vi "ECC_v3.vi"() -> ()   [LabVIEW 2019]
uses:
  state_machine.ctl
  <vilib>/DAQmx/write.llb/DAQmx Write (Analog Wfm 1Chan NSamp).vi
  <vilib>/DAQmx/create/channels.llb/DAQmx Create Channel (AO-Voltage-Basic).vi
  <vilib>/DAQmx/configure/timing.llb/DAQmx Timing (Use Waveform).vi
  <vilib>/DAQmx/miscellaneous.llb/DAQmx Fill In Error Info.vi
panel:
  in  "Use_DAC":bool
  out "AMP_status":bool
  in  "APS/APM":bool=TRUE
  in  "AMP address":tag="Dev1/port0/line0"
  in  "R&S/5181":bool=TRUE
  out "Pause, s":i32
  out "APS_off_status":bool=TRUE
  out "R&S_off_status":bool=TRUE
  out "Countdown":u32
  in  "Rep_delay":u32
  in  "Finite/Continuous":bool
  in  "ResumeSweep":bool
  in  "PauseSweep":bool
  in  "RF_off_rep":bool=TRUE
  in  "RF_off_set":bool
  in  "RF_off_cycle":bool
  in  "APS_off_rep":bool=TRUE
  in  "APS_off_set":bool
  in  "APS_off_cycle":bool
  in  "AbortSweep":bool
  in  "Check APS":bool
  in  "ON/OFF_APS":bool
  in  "Check R&S":bool
  in  "ON/OFF_RF":bool
  in  "Use_APS":bool
  out "DAC_status":bool
  out "RF_status":bool
  out "i_Current_repetition":i32
  out "N_Cycles_Created":i32
  out "i_Current_cycle":i32
  in  "M_repetitions":i32 min=0
  in  "Set_of_Cycles":T1(array[cluster])=[{"On/Off"=TRUE, "f0, MHz"=32.5, "fm, kHz"=1000, "A, mV"=20, "Waveform"=enum."triangle", "N_steps"=500, "T_sweep, s"=10.0, "N_sweeps"=5, "End_Wait, s"=0}, {"On/Off"=TRUE, "f0, MHz"=62.7, "fm, kHz"=400, "A, mV"=10, "Waveform"=enum."triangle", "N_steps"=500, "T_sweep, s"=10.0, "N_sweeps"=5, "End_Wait, s"=0}] {"End_Wait, s" step=1; "N_sweeps" min=0 step=1; "T_sweep, s" min=0.0 step=0.001 format="%#_6f"; "N_steps" min=0 step=1; "fm, kHz" step=1; "f0, MHz" min=0.0 step=0.001 format="%#_6f"}
  out "APS_status":bool
  in  "APS address":refnum<visa-resource-name>="COM3"
  in  "Init Devices":bool
  in  "Do Sweep":bool
  in  "Exit":bool
  in  "DAC channel":tag="Dev1/ao0"
  in  "RF address":string(combo)="19"
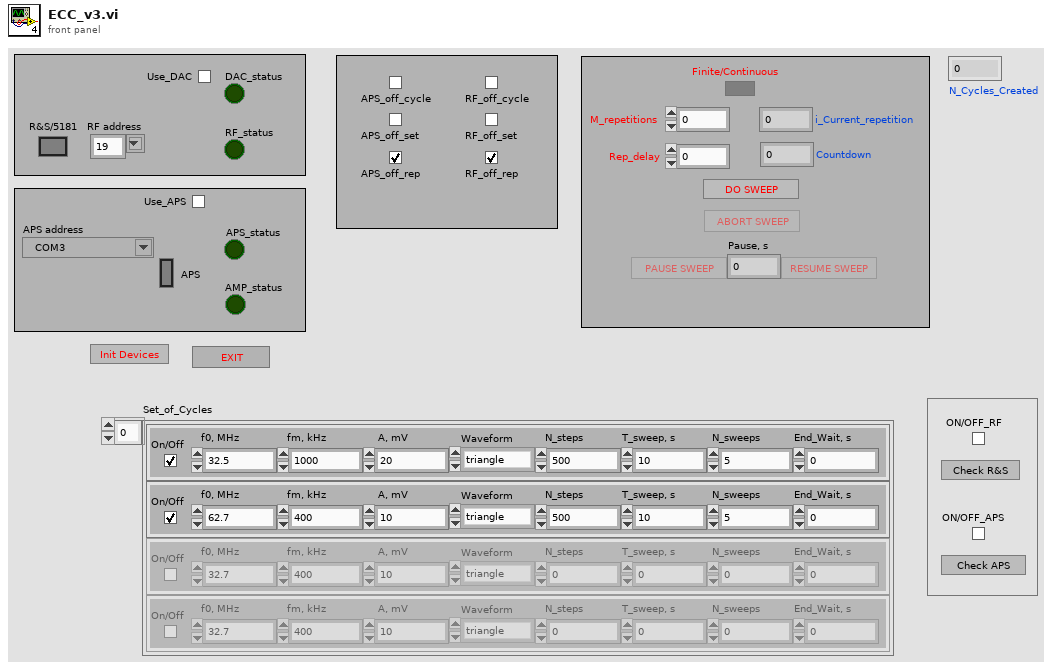
[diagram p1: front panel]
types:
  T1 = cluster{"On/Off":bool, "f0, MHz":dbl, "fm, kHz":i32, "A, mV":i32, "Waveform":enum16{"triangle", "saw_direct", "saw_invert", "sine"}, "N_steps":i32, "T_sweep, s":dbl, "N_sweeps":i32, "End_Wait, s":u32}[]
  T2 = typedef "state_machine.ctl" = enum16{"idle", "init_daq", "init_rf", "init_ps", "cycle_start", "get_wf", "rf_on", "rf_off", "rf_set", "ps_on", "ps_off", "daq_start", "daq_stop", "daq_wait", "daq_dt", "daq_v", "delay", "cycle_reset", "exit", "repetition_reset"}
  T3 = enum8{"Enabled", "Disabled", "Disabled and Grayed Out"}
  T4 = cluster{"On/Off":bool, "f0, MHz":dbl, "fm, kHz":i32, "A, mV":i32, "Waveform":enum16{"triangle", "saw_direct", "saw_invert", "sine"}, "N_steps":i32, "T_sweep, s":dbl, "N_sweeps":i32, "End_Wait, s":u32}
  T5 = enum16{"triangle", "saw_direct", "saw_invert", "sine"}
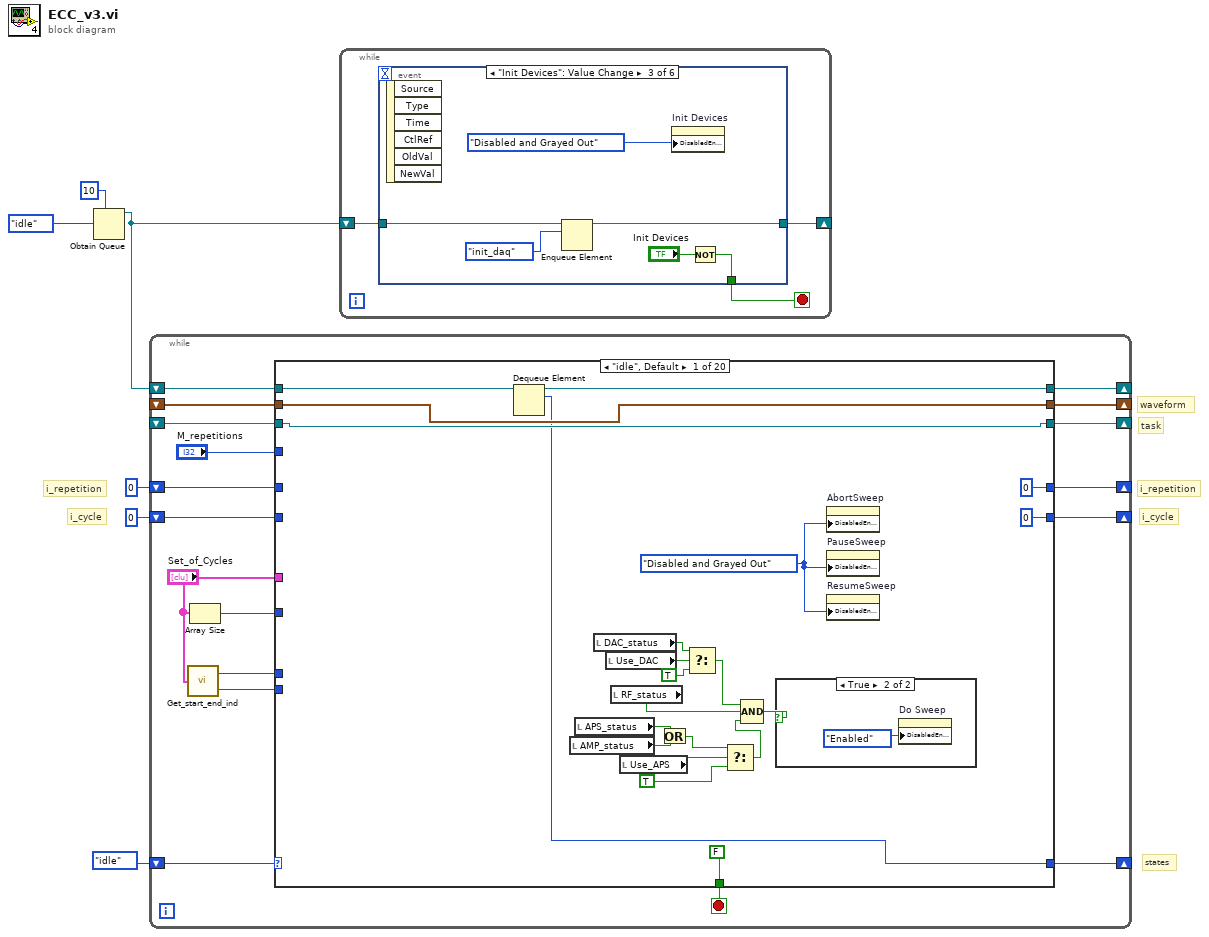
[diagram p0: block diagram]
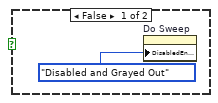
[diagram p2: hidden frame]
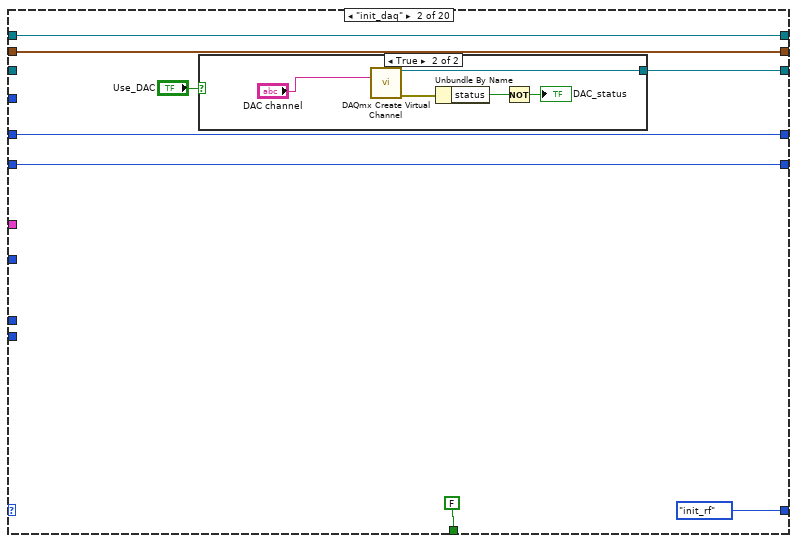
[diagram p3: hidden frame]
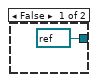
[diagram p4: hidden frame]
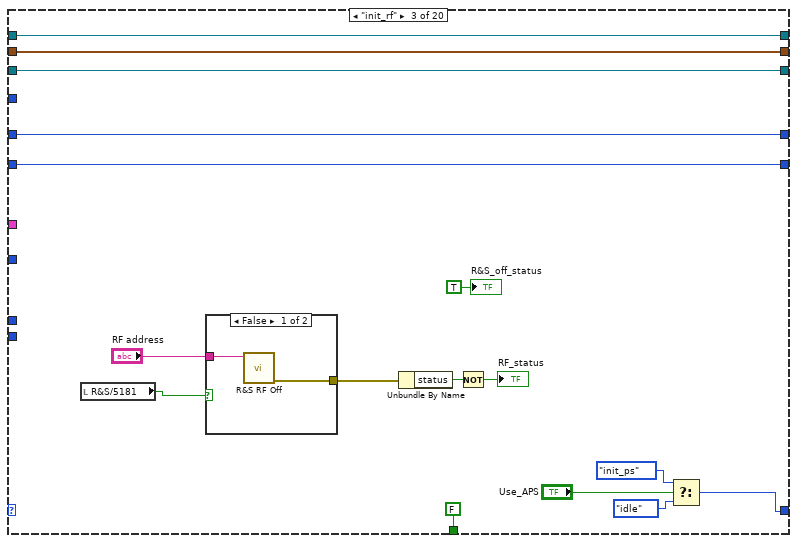
[diagram p5: hidden frame]
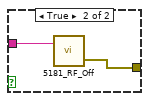
[diagram p6: hidden frame]
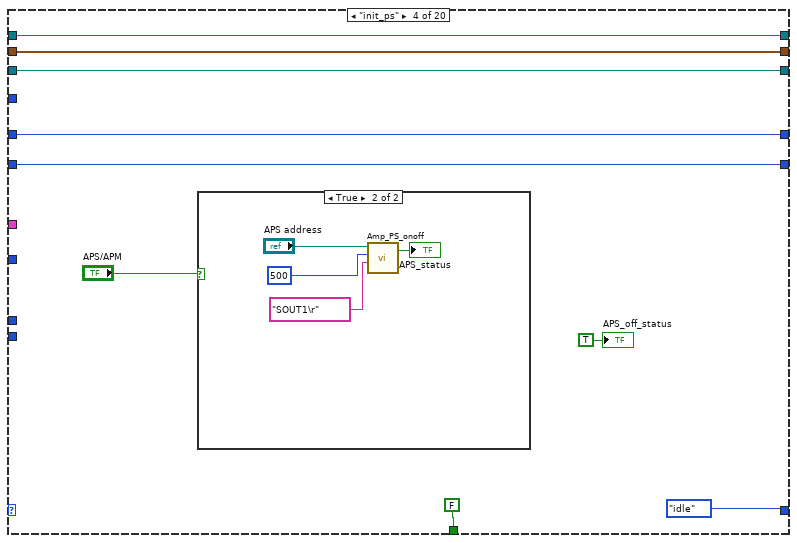
[diagram p7: hidden frame]
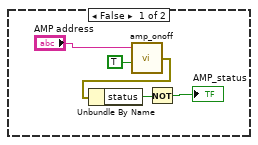
[diagram p8: hidden frame]
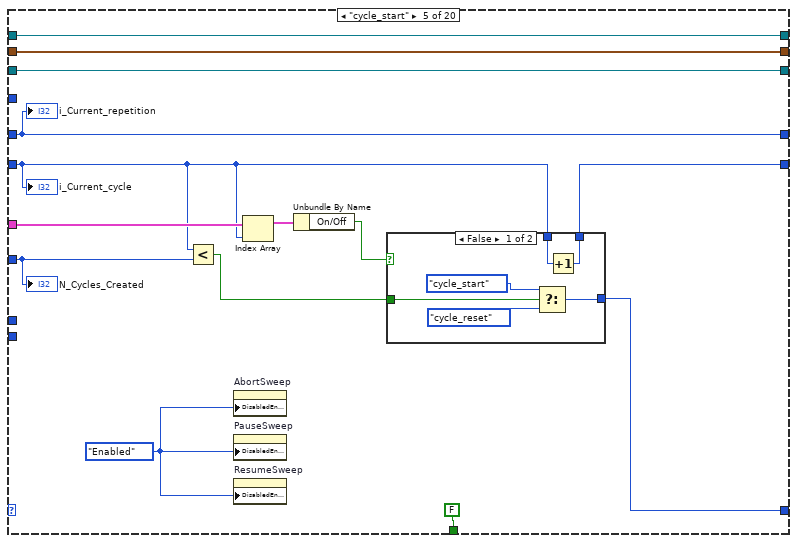
[diagram p9: hidden frame]
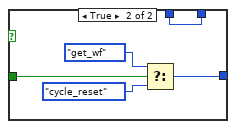
[diagram p10: hidden frame]
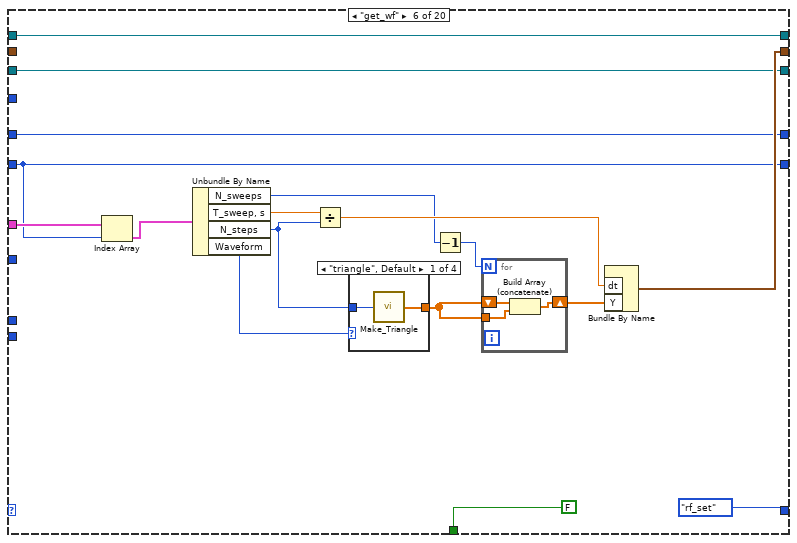
[diagram p11: hidden frame]
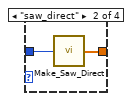
[diagram p12: hidden frame]
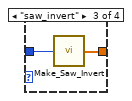
[diagram p13: hidden frame]
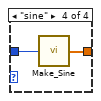
[diagram p14: hidden frame]
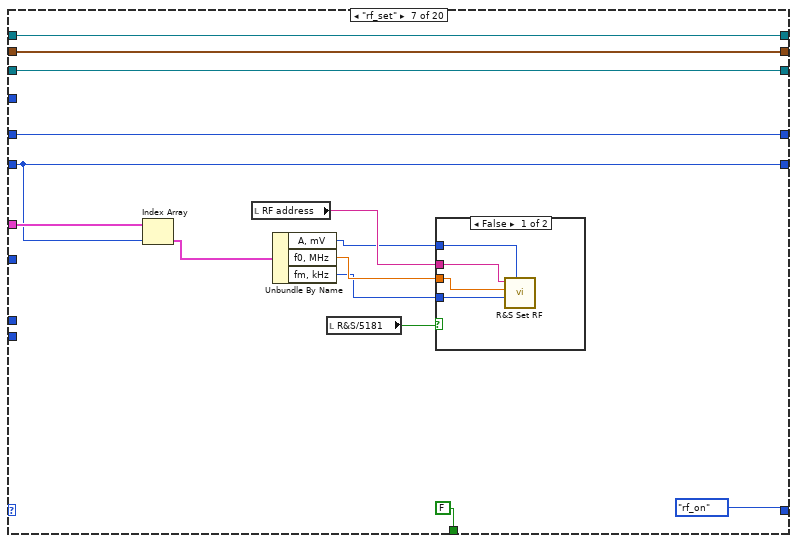
[diagram p15: hidden frame]
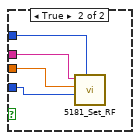
[diagram p16: hidden frame]
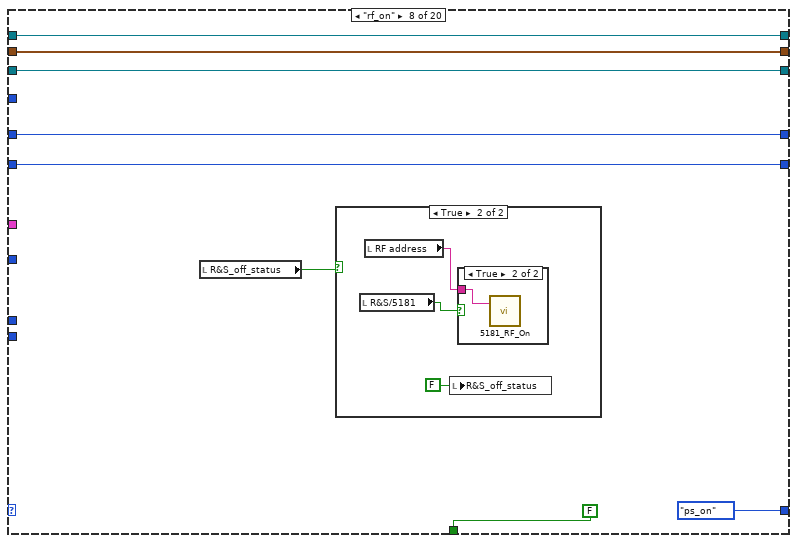
[diagram p17: hidden frame]
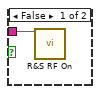
[diagram p19: hidden frame]
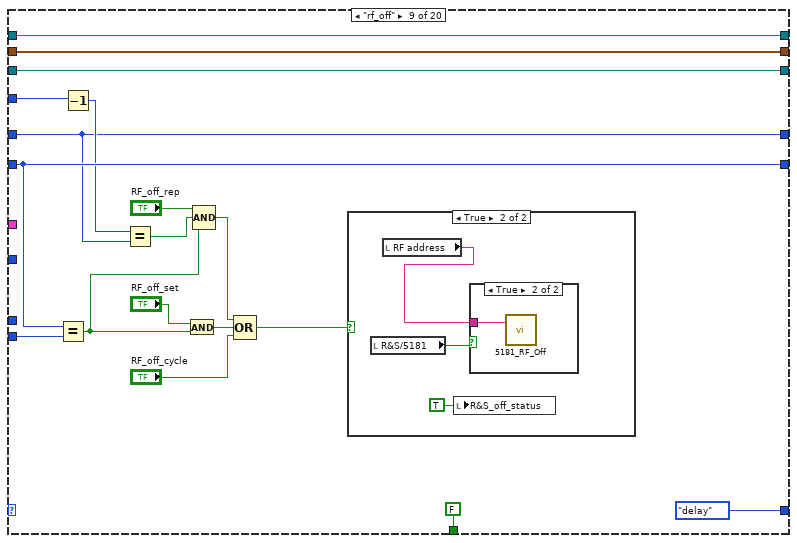
[diagram p20: hidden frame]
diagram:
  # "i_repetition"
  # "i_cycle"
  # "i_repetition"
  # "i_cycle"
  # "states"
  # "waveform"
  # "task"
  n1 = Obtain Queue(max queue size (-1, unlimited)=10, element data type=state_machine."idle") -> (queue out=w4:refnum<queue>)  [unwired: 3 in, 2 out]
  n2 = while {
    shift-right: [w19] -> _
    shift-left: state_machine."idle" -> [w24]
    shift-right: [w23] -> _
    shift-left: _ -> [w21]
    shift-right: [w22] -> _
    shift-left: _ -> [w20]
    shift-right: [w17] -> _
    shift-left: w4 -> [w18]
    shift-right: [w15] -> _
    shift-left: 0 -> [w14]
    shift-right: [w13] -> _
    shift-left: 0 -> [w12]
    stop <- w16 stop-if-true
    n3 = call "Get_start_end_ind.vi"("Set_of_Cycles"="Set_of_Cycles") -> ("start_ind"=w9:i32, "end_ind"=w8:i32)
    n4 = Array Size(array="Set_of_Cycles") -> (size(s)=w11:i32)
    n5 = case shown="\"idle\", Default" w24 {
      selector: w24 -> [_ _ _ _ _ _ _ _ _ _ _ _ _ _ _ _ _ _ w404 _]
      tunnel: [w45 w55 w77 w90 w103 w134 w163 w180 w203 w222 w243 w271 w283 w295 w307 w320 w336 w354 w401 w412] -> w23
      tunnel: "Set_of_Cycles" -> [_ _ _ _ w113 w141 w165 _ _ _ _ _ _ _ _ _ w333 _ _ _]
      tunnel: [w44 w54 w76 w89 w104 w135 w162 w181 w204 w221 w242 w270 w282 w294 w306 w321 w337 w353 w400 w413] -> w22
      tunnel: w21 -> [w45 _ w77 w90 w103 w134 w163 w180 w203 w222 w243 w272 w284 w296 w308 w322 w336 w354 w401 w412]
      tunnel: w20 -> [w44 w54 w76 w89 w104 _ w162 w181 w204 w221 w242 w270 w282 w294 w306 w321 w337 w353 w400 w413]
      tunnel: [w41 state_machine."init_rf" w67 state_machine."idle" w109 state_machine."rf_set" state_machine."rf_on" state_machine."ps_on" state_machine."delay" state_machine."daq_dt" state_machine."rf_off" state_machine."daq_wait" state_machine."ps_off" state_machine."daq_stop" state_machine."daq_v" state_machine."daq_start" state_machine."cycle_start" w352 w404 w408] -> w19
      tunnel: w18 -> [w43 w51 w74 w86 w102 w132 w160 w182 w205 w218 w239 w267 w279 w291 w303 w317 w338 w355 w403 w415]
      tunnel: [w42 w51 w74 w86 w102 w132 w160 w182 w205 w218 w239 w267 w279 w291 w303 w317 w338 w355 w403 w415] -> w17
      tunnel: [FALSE FALSE FALSE FALSE FALSE FALSE FALSE FALSE FALSE FALSE FALSE FALSE FALSE FALSE FALSE FALSE FALSE FALSE TRUE FALSE] -> w16
      tunnel: w11 -> [_ _ _ _ w105 _ _ _ _ _ _ _ _ _ _ _ _ _ _ _]
      tunnel: [0 w50 w73 w85 w108 w125 w158 w176 w199 w216 w237 w266 w278 w290 w302 w316 w328 0 w399 w414] -> w15
      tunnel: w14 -> [_ w50 w73 w85 w106 w125 w158 w176 w199 w216 w237 w266 w278 w290 w302 w316 w327 _ w399 w414]
      tunnel: [0 w49 w72 w84 w101 w127 w159 w179 w191 w217 w233 w265 w277 w289 w301 w315 w335 w349 w398 0] -> w13
      tunnel: w12 -> [_ w49 w72 w84 w101 w127 w159 w179 w191 w217 w233 w265 w277 w289 w301 w315 w335 w350 w398 _]
      tunnel: "M_repetitions" -> [_ _ _ _ _ _ _ _ w196 _ w235 _ _ _ _ _ _ w357 _ _]
      tunnel: w9 -> [_ _ _ _ _ _ _ _ _ _ _ _ _ _ _ _ _ _ _ _]
      tunnel: w8 -> [_ _ _ _ _ _ _ _ w200 _ w238 _ _ _ _ _ _ _ _ _]
      frame "idle", Default {
        w32 = T3."Disabled and Grayed Out" ("Disabled")
        n6 = Dequeue Element(queue=w43) -> (queue out=w42:refnum<queue>, element=w41:T2)  [unwired: 2 in, 2 out]
        n7 = local read "AMP_status"() -> (w30:bool)
        n8 = local read "APS_status"() -> (w31:bool)
        n9 = local read "DAC_status"() -> (w27:bool)
        n10 = local read "Use_DAC"() -> (w25:bool)
        n11 = local read "RF_status"() -> (w37:bool)
        n12 = local read "Use_APS"() -> (w36:bool)
        n13 = Or(x=w31, y=w30) -> (x .or. y?=w29:bool)
        n14 = Select(t=w27, s=w25, f=TRUE) -> (s? t:f=w28:bool)
        n15 = Select(t=w29, s=w36, f=TRUE) -> (s? t:f=w34:bool)
        n16 = Compound Arithmetic op=AND(w28, w37, w34) -> (w33:bool)
        n17 = case shown="True" w33 {
          frame False {
            n18 = property on="Do Sweep" class="Bool"("DisabledEnum"=T3."Disabled and Grayed Out" ("Disabled")) -> ()  [unwired: 2 in, 2 out]
          }
          frame True {
            n19 = property on="Do Sweep" class="Bool"("DisabledEnum"=T3."Enabled" ("Disabled")) -> ()  [unwired: 2 in, 2 out]
          }
        }
        n20 = property on="AbortSweep" class="Bool"("DisabledEnum"=w32) -> ()  [unwired: 2 in, 2 out]
        n21 = property on="PauseSweep" class="Bool"("DisabledEnum"=w32) -> ()  [unwired: 2 in, 2 out]
        n22 = property on="ResumeSweep" class="Bool"("DisabledEnum"=w32) -> ()  [unwired: 2 in, 2 out]
      }
      frame "init_daq" {
        n23 = case shown="True" "Use_DAC" {
          tunnel: [refnum<k21> refnum ("task out") w60] -> w55
          frame False {
          }
          frame True {
            n24 = call-poly <vilib>:"DAQmx Create Virtual Channel.vi"("physical channels"="DAC channel") -> ("task out"=w60:refnum<k21>, "error out"=w59:errorcluster)  [unwired: 13 in]
            n25 = Unbundle By Name(w59) -> ("status"=w58:bool)
            n26 = Not(x=w58) -> (.not. x?=→"DAC_status":bool)
          }
        }
      }
      frame "init_rf" {
        n27 = local read "R&S/5181"() -> (w62:bool)
        n28 = case shown="False" w62 {
          tunnel: "RF address" -> [w79 w81]
          tunnel: [w78 w80] -> w63
          frame False {
            n29 = call "R&S RF Off.vi"("address"=w79) -> ("error out"=w78:errorcluster)  [unwired: 5 in, 1 out]
          }
          frame True {
            n30 = call "5181_RF_Off.vi"("address"=w81) -> ("error out"=w80:errorcluster)  [unwired: 1 in, 1 out]
          }
        }
        n31 = Unbundle By Name(w63) -> ("status"=w70:bool)
        n32 = Not(x=w70) -> (.not. x?=→"RF_status":bool)
        n33 = Select(t=state_machine."init_ps", s="Use_APS", f=state_machine."idle") -> (s? t:f=w67:T2)
        "R&S_off_status" <- TRUE ("R&S_off_status")
      }
      frame "init_ps" {
        n34 = case shown="True" "APS/APM" {
          frame False {
            n35 = call "amp_onoff.vi"("amp_onoff"=TRUE, "AMP address"="AMP address") -> ("error out"=w93:errorcluster)  [unwired: 1 in]
            n36 = Unbundle By Name(w93) -> ("status"=w94:bool)
            n37 = Not(x=w94) -> (.not. x?=→"AMP_status":bool)
          }
          frame True {
            n38 = call "Amp_PS_onoff.vi"("On/Off Control"="SOUT1\r", "delay before read (ms)"=u32 500, "Amp PS address"="APS address") -> ("status"=→"APS_status":bool)  [unwired: 1 in, 1 out]
          }
        }
        "APS_off_status" <- TRUE ("APS_off_status")
      }
      frame "cycle_start" {
        w100 = T3."Enabled" ("Disabled")
        n39 = Less?(x=w106, y=w105) -> (x < y?=w110:bool)
        n40 = property on="AbortSweep" class="Bool"("DisabledEnum"=w100) -> ()  [unwired: 2 in, 2 out]
        n41 = property on="PauseSweep" class="Bool"("DisabledEnum"=w100) -> ()  [unwired: 2 in, 2 out]
        n42 = property on="ResumeSweep" class="Bool"("DisabledEnum"=w100) -> ()  [unwired: 2 in, 2 out]
        n43 = Index Array(array=w113, index=w106) -> (element=w112:T4)
        n44 = Unbundle By Name(w112) -> ("On/Off"=w111:bool)
        n45 = case shown="False" w111 {
          tunnel: w110 -> [w117 w123]
          tunnel: [w114 w122] -> w109
          tunnel: w106 -> [w119 w120]
          tunnel: [w118 w120] -> w108
          frame False {
            n46 = Select(t=state_machine."cycle_start", s=w117, f=state_machine."cycle_reset") -> (s? t:f=w114:T2)
            n47 = Increment(x=w119) -> (x+1=w118:i32)
          }
          frame True {
            n48 = Select(t=state_machine."get_wf", s=w123, f=state_machine."cycle_reset") -> (s? t:f=w122:T2)
          }
        }
        "N_Cycles_Created" <- w105
        "i_Current_cycle" <- w106
        "i_Current_repetition" <- w101
      }
      frame "get_wf" {
        n49 = Index Array(array=w141, index=w125) -> (element=w140:T4)
        n50 = Unbundle By Name(w140) -> ("N_sweeps"=w131:i32, "T_sweep, s"=w129:dbl, "N_steps"=w128:i32, "Waveform"=w130:T5)
        n51 = Divide(x=w129, y=w128) -> (x/y=w137:dbl)
        n52 = case shown="\"triangle\", Default" w130 {
          tunnel: w128 -> [w146 w148 w150 w152]
          tunnel: [w145 w147 w149 w151] -> w138
          frame "triangle", Default {
            n53 = call "Make_Triangle.vi"("N_steps_1"=w146) -> ("TriangleWaveform"=w145:dbl[])
          }
          frame "saw_direct" {
            n54 = call "Make_Saw_Direct.vi"("N_steps_1"=w148) -> ("SawDirectWaveform"=w147:dbl[])
          }
          frame "saw_invert" {
            n55 = call "Make_Saw_Invert.vi"("N_steps_1"=w150) -> ("SawInvertWaveform"=w149:dbl[])
          }
          frame "sine" {
            n56 = call "Make_Sine.vi"("N_steps_1"=w152) -> ("SineWaveform"=w151:dbl[])
          }
        }
        n57 = Decrement(x=w131) -> (x-1=w136:i32)
        n58 = for {
          N: w136 -> [_]
          shift-right: [w142] -> w139
          shift-left: w138 -> [w144]
          tunnel: w138 -> [w143]
          n59 = Build Array (concatenate)(w144, w143) -> (w142:dbl[])
        }
        n60 = Bundle By Name("dt"=w137, "Y"=w139) -> (w135:waveform(dbl))  [unwired: 1 in]
      }
      frame "rf_set" {
        n61 = Index Array(array=w165, index=w158) -> (element=w164:T4)
        n62 = local read "RF address"() -> (w166:string)
        n63 = Unbundle By Name(w164) -> ("A, mV"=w157:i32, "f0, MHz"=w156:dbl, "fm, kHz"=w155:i32)
        n64 = local read "R&S/5181"() -> (w153:bool)
        n65 = case shown="False" w153 {
          tunnel: w166 -> [w170 w174]
          tunnel: w157 -> [w169 w173]
          tunnel: w156 -> [w168 w172]
          tunnel: w155 -> [w167 w171]
          frame False {
            n66 = call "R&S Set RF.vi"("amplitude (mV)"=w169, "modulation (kHz)"=w167, "center frequency (MHz)"=w168, "address"=w170) -> ()  [unwired: 3 in, 2 out]
          }
          frame True {
            n67 = call "5181_Set_RF.vi"("address"=w174, "center frequency (MHz)"=w172, "modulation (kHz)"=w171, "amplitude (mV)"=w173) -> ()  [unwired: 1 in, 2 out]
          }
        }
      }
      frame "rf_on" {
        n68 = local read "R&S_off_status"() -> (w175:bool)
        n69 = case shown="True" w175 {
          frame False {
          }
          frame True {
            n70 = local read "R&S/5181"() -> (w183:bool)
            n71 = local read "RF address"() -> (w185:string)
            n72 = local write "R&S_off_status"(FALSE ("R&S_off_status")) -> ()
            n73 = case shown="True" w183 {
              tunnel: w185 -> [w186 w187]
              frame False {
                n74 = call "R&S RF On.vi"("address"=w186) -> ()  [unwired: 5 in, 2 out]
              }
              frame True {
                n75 = call "5181_RF_On.vi"("address"=w187) -> ()  [unwired: 1 in, 2 out]
              }
            }
          }
        }
      }
      frame "rf_off" {
        n76 = Equal?(x=w199, y=w200) -> (x = y?=w188:bool)
        n77 = Decrement(x=w196) -> (x-1=w192:i32)
        n78 = Equal?(x=w192, y=w191) -> (x = y?=w189:bool)
        n79 = And(x="RF_off_set", y=w188) -> (x .and. y?=w195:bool)
        n80 = Compound Arithmetic op=AND("RF_off_rep", w189, w188) -> (w193:bool)
        n81 = Compound Arithmetic op=OR(w193, w195, "RF_off_cycle") -> (w197:bool)
        n82 = case shown="True" w197 {
          frame False {
          }
          frame True {
            n83 = local read "R&S/5181"() -> (w206:bool)
            n84 = local read "RF address"() -> (w208:string)
            n85 = local write "R&S_off_status"(TRUE ("R&S_off_status")) -> ()
            n86 = case shown="True" w206 {
              tunnel: w208 -> [w209 w210]
              frame False {
                n87 = call "R&S RF Off.vi"("address"=w209) -> ()  [unwired: 5 in, 2 out]
              }
              frame True {
                n88 = call "5181_RF_Off.vi"("address"=w210) -> ()  [unwired: 1 in, 2 out]
              }
            }
          }
        }
      }
      frame "ps_on" {
        n89 = local read "APS_status"() -> (w211:bool)
        n90 = local read "APS_status"() -> (w213:bool)
        n91 = local read "APS_off_status"() -> (w215:bool)
        n92 = Or(x=w213, y=w211) -> (x .or. y?=w212:bool)
        n93 = And(x=w212, y=w215) -> (x .and. y?=w214:bool)
        n94 = case shown="True" w214 {
          frame False {
          }
          frame True {
            n95 = local read "APS/APM"() -> (w223:bool)
            n96 = case shown="True" w223 {
              frame False {
                n97 = local read "AMP address"() -> (w225:tag)
                n98 = call "amp_onoff.vi"("amp_onoff"=TRUE, "AMP address"=w225) -> ()  [unwired: 1 in, 1 out]
              }
              frame True {
                n99 = local read "APS address"() -> (w227:refnum<visa-resource-name>)
                n100 = call "Amp_PS_onoff.vi"("On/Off Control"="SOUT0\r", "delay before read (ms)"=u32 500, "Amp PS address"=w227) -> ()  [unwired: 1 in, 2 out]
              }
            }
            n101 = local write "APS_off_status"(FALSE ("APS_off_status")) -> ()
          }
        }
      }
      frame "ps_off" {
        n102 = Decrement(x=w235) -> (x-1=w234:i32)
        n103 = local read "APS_status"() -> (w231:bool)
        n104 = local read "APS_status"() -> (w232:bool)
        n105 = Or(x=w232, y=w231) -> (x .or. y?=w230:bool)
        n106 = case shown="True" w230 {
          selector: w230 -> [w244 _]
          tunnel: w238 -> [_ w256]
          tunnel: w237 -> [_ w255]
          tunnel: [w244 w250] -> w236
          tunnel: w234 -> [_ w246]
          tunnel: w233 -> [_ w247]
          frame False {
          }
          frame True {
            n107 = Equal?(x=w246, y=w247) -> (x = y?=w252:bool)
            n108 = Equal?(x=w255, y=w256) -> (x = y?=w245:bool)
            n109 = Compound Arithmetic op=AND("APS_off_rep", w252, w245) -> (w249:bool)
            n110 = And(x="APS_off_set", y=w245) -> (x .and. y?=w251:bool)
            n111 = Compound Arithmetic op=OR(w249, w251, "APS_off_cycle") -> (w250:bool)
          }
        }
        n112 = case shown="True" w236 {
          frame False {
          }
          frame True {
            n113 = local read "APS/APM"() -> (w257:bool)
            n114 = case shown="True" w257 {
              frame False {
                n115 = local read "AMP address"() -> (w259:tag)
                n116 = call "amp_onoff.vi"("amp_onoff"=FALSE, "AMP address"=w259) -> ()  [unwired: 1 in, 1 out]
              }
              frame True {
                n117 = local read "APS address"() -> (w261:refnum<visa-resource-name>)
                n118 = call "Amp_PS_onoff.vi"("On/Off Control"="SOUT1\r", "delay before read (ms)"=u32 500, "Amp PS address"=w261) -> ()  [unwired: 1 in, 2 out]
              }
            }
            n119 = local write "APS_off_status"(TRUE ("APS_off_status")) -> ()
          }
        }
      }
      frame "daq_start" {
        n120 = local read "Use_DAC"() -> (w264:bool)
        n121 = case shown="True" w264 {
          tunnel: w272 -> [w273 w275]
          tunnel: [w273 w274] -> w271
          frame False {
          }
          frame True {
            n122 = call <vilib>:"DAQmx Start Task.vi"("task/channels in"=w275) -> ("task out"=w274:refnum<k21>)  [unwired: 13 in, 1 out]
          }
        }
      }
      frame "daq_stop" {
        n123 = local read "Use_DAC"() -> (w276:bool)
        n124 = case shown="True" w276 {
          tunnel: w284 -> [w285 w287]
          tunnel: [w285 w286] -> w283
          frame False {
          }
          frame True {
            n125 = call <vilib>:"DAQmx Stop Task.vi"("task/channels in"=w287) -> ("task out"=w286:refnum<k21>)  [unwired: 13 in, 1 out]
          }
        }
      }
      frame "daq_wait" {
        n126 = local read "Use_DAC"() -> (w288:bool)
        n127 = case shown="True" w288 {
          tunnel: w296 -> [w297 w299]
          tunnel: [w297 w298] -> w295
          frame False {
          }
          frame True {
            n128 = call <vilib>:"DAQmx Wait Until Done.vi"("task/channels in"=w299) -> ("task out"=w298:refnum<k21>)  [unwired: 13 in, 1 out]
          }
        }
      }
      frame "daq_dt" {
        n129 = local read "Use_DAC"() -> (w300:bool)
        n130 = case shown="True" w300 {
          tunnel: w308 -> [w309 w313]
          tunnel: [w309 w312] -> w307
          tunnel: w306 -> [_ w311]
          frame False {
          }
          frame True {
            w310 = 10178 items=["Finite Samples"=10178, "Continuous Samples"=10123, "Hardware Timed Single Point"=12522] ("sample mode")
            n131 = call-poly <vilib>:"DAQmx Timing.vi"("task/channels in"=w313, "sample mode"=w310, "waveform"=w311) -> ("task out"=w312:refnum<k21>)  [unwired: 11 in, 1 out]
          }
        }
      }
      frame "daq_v" {
        n132 = local read "Use_DAC"() -> (w314:bool)
        n133 = case shown="True" w314 {
          tunnel: w322 -> [w323 w326]
          tunnel: w321 -> [_ w325]
          tunnel: [w323 w324] -> w320
          frame False {
          }
          frame True {
            n134 = call-poly <vilib>:"DAQmx Write.vi"("task/channels in"=w326, "data"=w325) -> ("task out"=w324:refnum<k21>)  [unwired: 11 in, 2 out]
          }
        }
      }
      frame "delay" {
        # "iterate cycle"
        n135 = Increment(x=w327) -> (x+1=w328:i32)
        n136 = Index Array(array=w333, index=w327) -> (element=w334:T4)
        n137 = Unbundle By Name(w334) -> ("End_Wait, s"=w331:u32)
        n138 = Equal To 0?(x=w331) -> (x = 0?=w332:bool)
        n139 = case shown="True" w332 {
          tunnel: w331 -> [w339 _]
          frame False {
            n140 = Multiply(x=u32 1000 ("y"), y=w339) -> (x*y=w341:u32)
            n141 = Wait (ms)(milliseconds to wait=w341) -> ()  [unwired: 1 out]
          }
          frame True {
          }
        }
      }
      frame "cycle_reset" {
        # "iterate repetition"
        n142 = Increment(x=w350) -> (x+1=w342:i32)
        n143 = case shown="True" "PauseSweep" {
          selector: "PauseSweep" -> [w369 _]
          tunnel: [w369 w370] -> w346
          frame False {
          }
          frame True {
            n144 = Tick Count (ms)() -> (millisecond timer value=w371:u32)
            n145 = while {
              tunnel: w371 -> [w377]
              tunnel: ["ResumeSweep"] -> w370
              stop <- "ResumeSweep" stop-if-true
              n146 = Tick Count (ms)() -> (millisecond timer value=w378:u32)
              n147 = Subtract(x=w378, y=w377) -> (x-y=w376:u32)
              n148 = Divide(x=w376, y=u32 1000) -> (x/y=w374:dbl)
              n149 = To Long Integer(number=w374) -> (32bit integer=→"Pause, s":i32)
            }
          }
        }
        n150 = Less?(x=w342, y=w357) -> (x < y?=w351:bool)
        n151 = Or(x="AbortSweep", y="PauseSweep") -> (x .or. y?=w343:bool)
        n152 = case shown="False" "AbortSweep" {
          tunnel: [w387 state_machine."idle"] -> w352
          tunnel: w351 -> [w386 _]
          tunnel: w342 -> [w385 _]
          tunnel: [w385 0] -> w349
          frame False {
            n153 = Select(t=state_machine."cycle_start", s=w386, f=state_machine."repetition_reset") -> (s? t:f=w387:T2)
          }
          frame True {
            w391 = T3."Enabled" ("Disabled")
            n154 = property on="Check APS" class="Bool"("DisabledEnum"=w391) -> ()  [unwired: 2 in, 2 out]
            n155 = property on="Check R&S" class="Bool"("DisabledEnum"=w391) -> ()  [unwired: 2 in, 2 out]
          }
        }
        n156 = local read "APS_status"() -> (w344:bool)
        n157 = And(x=w343, y=w344) -> (x .and. y?=w345:bool)
        n158 = case shown="True" w343 {
          frame False {
          }
          frame True {
            n159 = local write "R&S_off_status"(TRUE ("R&S_off_status")) -> ()
            n160 = local read "RF address"() -> (w380:string)
            n161 = call "R&S RF Off.vi"("address"=w380) -> ()  [unwired: 5 in, 2 out]
          }
        }
        n162 = case shown="True" w346 {
          frame False {
          }
          frame True {
            n163 = local read "R&S_off_status"() -> (w364:bool)
            n164 = case shown="False" w364 {
              frame False {
                n165 = local read "RF address"() -> (w368:string)
                n166 = call "R&S RF On.vi"("address"=w368) -> ()  [unwired: 5 in, 2 out]
              }
              frame True {
              }
            }
            n167 = local write "Pause, s"(0 ("Pause, s")) -> ()
            n168 = local read "APS_off_status"() -> (w362:bool)
            n169 = local read "APS_status"() -> (w363:bool)
            n170 = Not(x=w362) -> (.not. x?=w361:bool)
            n171 = And(x=w363, y=w361) -> (x .and. y?=w360:bool)
            n172 = case shown="True" w360 {
              frame False {
              }
              frame True {
                n173 = local read "APS address"() -> (w365:refnum<visa-resource-name>)
                n174 = call "Amp_PS_onoff.vi"("On/Off Control"="SOUT0\r", "delay before read (ms)"=u32 50, "Amp PS address"=w365) -> ()  [unwired: 1 in, 2 out]
              }
            }
          }
        }
        n175 = case shown="True" w345 {
          frame False {
          }
          frame True {
            n176 = local read "APS address"() -> (w382:refnum<visa-resource-name>)
            n177 = local write "APS_off_status"(TRUE ("APS_off_status")) -> ()
            n178 = call "Amp_PS_onoff.vi"("On/Off Control"="SOUT1\r", "delay before read (ms)"=u32 500, "Amp PS address"=w382) -> ()  [unwired: 1 in, 2 out]
          }
        }
      }
      frame "exit" {
        w393 = FALSE ("DAC_status")
        n179 = local read "APS address"() -> (w396:refnum<visa-resource-name>)
        n180 = local read "Use_APS"() -> (w397:bool)
        n181 = local read "RF address"() -> (w395:string)
        n182 = case shown="False" w397 {
          tunnel: w396 -> [_ w405]
          frame False {
          }
          frame True {
            n183 = call "Amp_PS_onoff.vi"("On/Off Control"="SOUT1\r", "delay before read (ms)"=u32 50, "Amp PS address"=w405) -> ()  [unwired: 1 in, 2 out]
          }
        }
        n184 = call "R&S RF Off.vi"("address"=w395) -> ()  [unwired: 5 in, 2 out]
        n185 = property on="Init Devices" class="Bool"("DisabledEnum"=T3."Enabled" ("Disabled")) -> ()  [unwired: 2 in, 2 out]
        n186 = local write "DAC_status"(w393) -> ()
        n187 = local write "RF_status"(w393) -> ()
        n188 = local write "APS_status"(w393) -> ()
      }
      frame "repetition_reset" {
        n189 = case shown="True" "Finite/Continuous" {
          tunnel: [state_machine."idle" state_machine."cycle_start"] -> w408
          frame False {
          }
          frame True {
            n190 = Tick Count (ms)() -> (millisecond timer value=w418:u32)
            n191 = while {
              tunnel: w418 -> [w425]
              tunnel: "Rep_delay" -> [w421]
              stop <- w423 stop-if-true
              w420 = u32 1000 ("y")
              n192 = Tick Count (ms)() -> (millisecond timer value=w426:u32)
              n193 = Subtract(x=w426, y=w425) -> (x-y=w427:u32)
              n194 = Divide(x=w427, y=w420) -> (x/y=w428:dbl)
              n195 = Wait (ms)(milliseconds to wait=w420) -> ()  [unwired: 1 out]
              n196 = To Long Integer(number=w428) -> (32bit integer=w422:i32)
              n197 = Subtract(x=w421, y=w422) -> (x-y=w424:u32)
              "Countdown" <- w424
              n198 = Less Or Equal To 0?(x=w424) -> (x <= 0?=w423:bool)
            }
          }
        }
      }
    }
  }
  n199 = while {
    shift-right: [w429] -> _
    shift-left: w4 -> [w430]
    stop <- w431 stop-if-true
    n200 = event shown="[2] \"Init Devices\": Value Change" {
      selector: _ -> [_ _ _ _ _ _]
      dyn-events: _ -> [_ _ _ _ _ _]
      timeout: _ -> [_ _ _ _ _ _]
      tunnel: [_ "Exit" w441 w447 w454 w467] -> w431
      tunnel: w430 -> [w432 w435 w440 w446 w451 w464]
      tunnel: [w432 w434 w439 w445 w451 w464] -> w429
      event Timeout {
        n201 = event-data() -> ()  [unwired: 1 in, 3 out]
      }
      event "Exit": Value Change {
        n202 = event-data() -> ()  [unwired: 1 in, 6 out]
        n203 = Enqueue Element(queue=w435, element=state_machine."exit") -> (queue out=w434:refnum<queue>)  [unwired: 2 in, 2 out]
      }
      event "Init Devices": Value Change {
        n204 = event-data() -> ()  [unwired: 1 in, 6 out]
        n205 = Enqueue Element(queue=w440, element=state_machine."init_daq") -> (queue out=w439:refnum<queue>)  [unwired: 2 in, 2 out]
        n206 = property on="Init Devices" class="Bool"("DisabledEnum"=T3."Disabled and Grayed Out" ("Disabled")) -> ()  [unwired: 2 in, 2 out]
        n207 = Not(x="Init Devices") -> (.not. x?=w441:bool)
      }
      event "Do Sweep": Value Change {
        w443 = T3."Disabled and Grayed Out" ("Disabled")
        n208 = event-data() -> ()  [unwired: 1 in, 6 out]
        n209 = Enqueue Element(queue=w446, element=state_machine."cycle_start") -> (queue out=w445:refnum<queue>)  [unwired: 2 in, 2 out]
        n210 = Not(x="Do Sweep") -> (.not. x?=w447:bool)
        n211 = property on="Check R&S" class="Bool"("DisabledEnum"=w443) -> ()  [unwired: 2 in, 2 out]
        n212 = property on="Check APS" class="Bool"("DisabledEnum"=w443) -> ()  [unwired: 2 in, 2 out]
      }
      event "Check R&S": Value Change {
        n213 = event-data() -> ()  [unwired: 1 in, 6 out]
        n214 = local read "RF address"() -> (w452:string)
        n215 = case shown="True" "ON/OFF_RF" {
          tunnel: w452 -> [w456 w460]
          tunnel: "R&S/5181" -> [w455 w459]
          frame False {
            n216 = case shown="True" w455 {
              tunnel: w456 -> [w457 w458]
              frame False {
                n217 = call "R&S RF Off.vi"("address"=w457) -> ()  [unwired: 5 in, 2 out]
              }
              frame True {
                n218 = call "5181_RF_Off.vi"("address"=w458) -> ()  [unwired: 1 in, 2 out]
              }
            }
          }
          frame True {
            n219 = case shown="False" w459 {
              tunnel: w460 -> [w461 w462]
              frame False {
                n220 = call "R&S RF On.vi"("address"=w461) -> ()  [unwired: 5 in, 2 out]
              }
              frame True {
                n221 = call "5181_RF_On.vi"("address"=w462) -> ()  [unwired: 1 in, 2 out]
              }
            }
          }
        }
        n222 = Not(x="Check R&S") -> (.not. x?=w454:bool)
      }
      event "Check APS": Value Change {
        n223 = event-data() -> ()  [unwired: 1 in, 6 out]
        n224 = local read "APS address"() -> (w465:refnum<visa-resource-name>)
        n225 = case shown="False" "ON/OFF_APS" {
          tunnel: w465 -> [w468 w471]
          frame False {
            n226 = call "Amp_PS_onoff.vi"("On/Off Control"="SOUT1\r", "delay before read (ms)"=u32 50, "Amp PS address"=w468) -> ()  [unwired: 1 in, 2 out]
          }
          frame True {
            n227 = call "Amp_PS_onoff.vi"("On/Off Control"="SOUT0\r", "delay before read (ms)"=u32 50, "Amp PS address"=w471) -> ()  [unwired: 1 in, 2 out]
          }
        }
        n228 = Not(x="Check APS") -> (.not. x?=w467:bool)
      }
    }
  }
